vi "Init.vi"(8 "error in (no error)":errorcluster, 11 "Insite in":refnum<class "Insight.lvclass">) -> (0 "error out":errorcluster, 3 "Insite out":refnum<class "Insight.lvclass">)   [LabVIEW 2015, in "Insight.lvclass"]
uses:
  Insight.lvclass
  Insight.lvclass/Insight.ctl
  <vilib>/Utility/file.llb/Read Delimited Spreadsheet (DBL).vi
  Laser.lvclass
panel:
  in  "file path (dialog if empty)":path=path "\\\\192.168.1.100\\data/DVV.txt"
  out "Waveform Graph 2":i32[](graph)
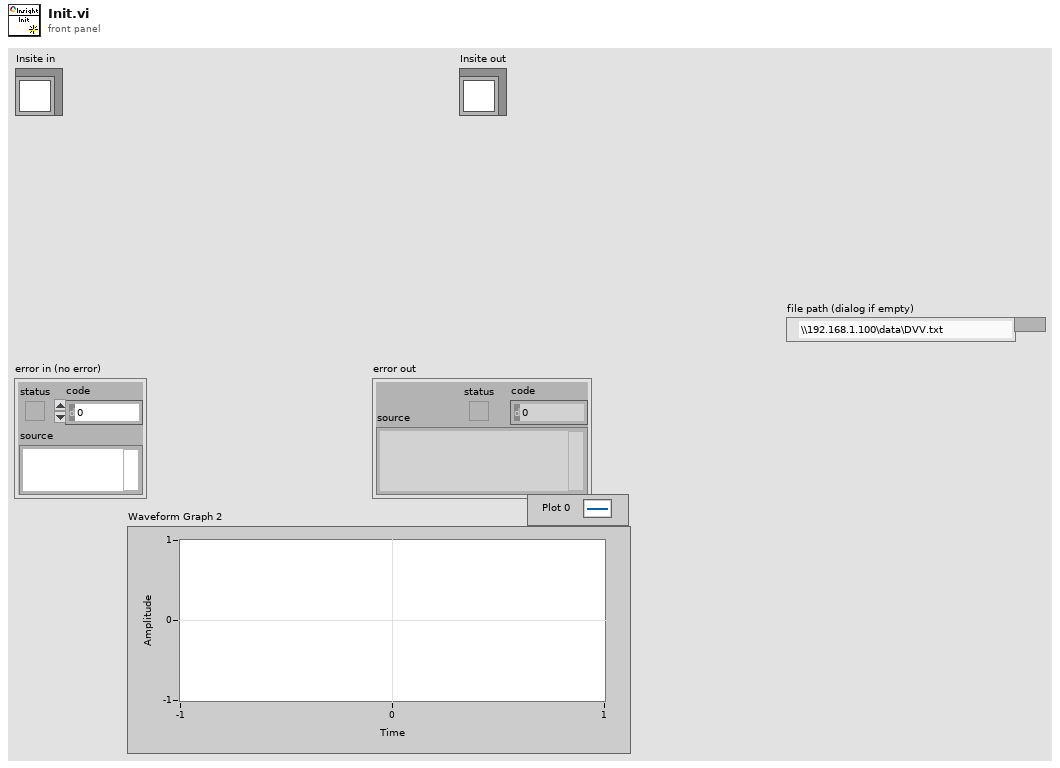
[diagram p1: front panel]
types:
  T1 = typedef "Telnet Session.ctl" = refnum<k1>
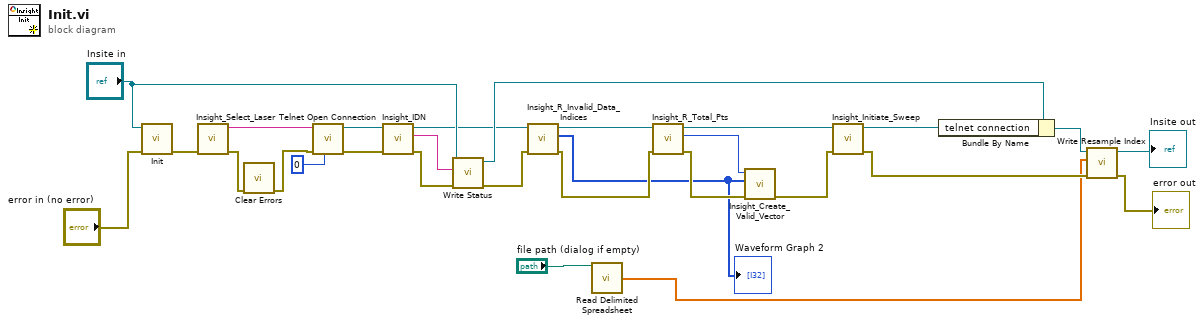
[diagram p0: block diagram]
diagram:
  n1 = call-parent "Init.vi"("error in (no error)"="error in (no error)", "Laser in"="Insite in") -> ("error out"=w27:errorcluster)  [unwired: 8 in, 1 out]
  n2 = call "Insight_Select_Laser.vi"("error in (no error)"=w27) -> ("error out"=w23:errorcluster, "IP address"=w26:string)  [unwired: 9 in]
  n3 = call <vilib>:"Clear Errors.vi"("error in (no error)"=w23) -> ("error out"=w24:errorcluster)  [unwired: 5 in, 1 out]
  n4 = call "Telnet Open Connection.vi"("local port"=u16 0, "error in (no error)"=w24, "address"=w26) -> ("error out"=w21:errorcluster, "telnet connection"=w22:T1)  [unwired: 7 in]
  n5 = call "Insight_IDN.vi"("error in (no error)"=w21, "telnet connection"=w22) -> ("error out"=w19:errorcluster, "*IDN?"=w20:string, "telnet  connection out"=w16:T1)  [unwired: 7 in]
  n6 = call-dynamic "Write Status.vi"("error in (no error)"=w19, "Status"=w20, "Laser in"="Insite in") -> ("error out"=w15:errorcluster, "Laser out"=w17:refnum<class "Insight.lvclass">)  [unwired: 7 in]
  n7 = call "Insight_R_Invalid_Data_Indices.vi"("error in (no error)"=w15, "telnet connection"=w16) -> ("error out"=w10:errorcluster, "Invalid Data Indices"=w3:i32[], "telnet  connection out"=w11:T1)  [unwired: 6 in, 1 out]
  "Waveform Graph 2" <- w3
  n8 = call-poly <vilib>:"Read Delimited Spreadsheet.vi"("file path (dialog if empty)"="file path (dialog if empty)") -> ("first row"=w1:dbl[])  [unwired: 9 in, 5 out]
  n9 = call "Insight_R_Total_Pts.vi"("error in (no error)"=w10, "telnet connection"=w11) -> ("error out"=w9:errorcluster, "Total Points"=w4:u32, "telnet  connection out"=w8:T1)  [unwired: 6 in, 1 out]
  n10 = call "Insight_Create_Valid_Vector.vi"("error in (no error)"=w9, "Invalid Data Indices"=w3, "total data length"=w4) -> ("error out"=w6:errorcluster)  [unwired: 7 in, 1 out]
  n11 = call "Insight_Initiate_Sweep.vi"("error in (no error)"=w6, "telnet connection"=w8) -> ("error out"=w5:errorcluster, "telnet  connection out"=w7:T1)  [unwired: 7 in, 1 out]
  n12 = Bundle By Name(cluster=w17, "telnet connection"=w7) -> (w14:refnum<class "Insight.lvclass">)
  n13 = call-dynamic "Write Resample Index.vi"("error in (no error)"=w5, "Resample Index"=w1, "Laser in"=w14) -> ("error out"=→"error out":errorcluster, "Laser out"=→"Insite out":refnum<class "Insight.lvclass">)  [unwired: 7 in]
